vi "FG COP Info.vi"(1 "FG Action (Read)":T1, 2 "COP Info in":T2) -> (0 "COP Info out":T2)   [LabVIEW 2011]
uses:
  cRIO/Functional Global Variables/Actions for FG's.ctl
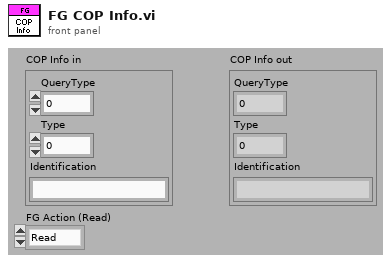
[diagram p1: front panel]
types:
  T1 = typedef "Actions for FG's.ctl" = enum16{"Read", "Write"}
  T2 = cluster{"QueryType":u8, "Type":u16, "Identification":string}
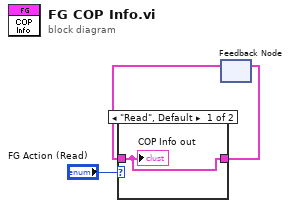
[diagram p0: block diagram]
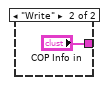
[diagram p2: hidden frame]
diagram:
  n1 = feedback #1() -> (w2:T2)  [unwired: 1 in]
  n2 = case shown="\"Read\", Default" "FG Action (Read)" {
    tunnel: w2 -> [w4 _]
    tunnel: [w4 "COP Info in"] -> w3
    frame "Read", Default {
      "COP Info out" <- w4
    }
    frame "Write" {
    }
  }
  n3 = feedback-in #1(w3) -> ()
